vi "Wave2D_Solve QU.vi"(9 "LU of Q":T1, 10 "Q":T3, 11 "U":dbl[][](array[numeric])) -> (0 "error":i32, 3 "Q\\U":dbl[][](array[numeric]))   [LabVIEW 2017, in "NI_PDE.lvlib"]
uses:
  <vilib>/gmath/NI_PDE.lvlib
  <vilib>/Analysis/Matrix/Datatypes/RealMatrix.ctl
  <vilib>/Analysis/7linalg.llb/Solve Linear Equations (multiple right hand).vi
  <vilib>/Analysis/NI_AALPro.lvlib
  <vilib>/Analysis/Matrix/NI_Matrix.lvlib
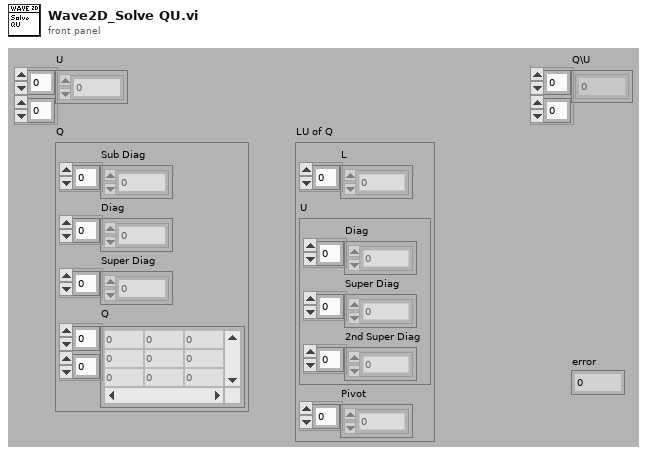
[diagram p1: front panel]
types:
  T1 = cluster{"L":dbl[], "U":cluster{"Diag":dbl[], "Super Diag":dbl[], "2nd Super Diag":dbl[]}, "Pivot":i32[]}
  T2 = typedef "NI_Matrix.lvlib/RealMatrix.ctl" = dbl[][]
  T3 = cluster{"Sub Diag":dbl[], "Diag":dbl[], "Super Diag":dbl[], "Q":T2}
  T4 = cluster{"Diag":dbl[], "Super Diag":dbl[], "2nd Super Diag":dbl[]}
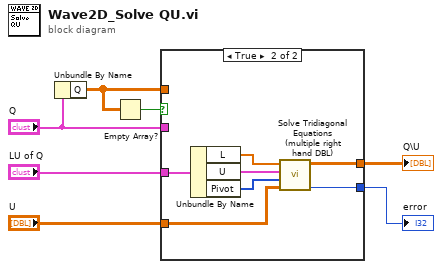
[diagram p0: block diagram]
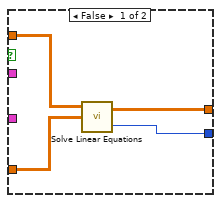
[diagram p2: hidden frame]
diagram:
  n1 = Unbundle By Name("Q") -> ("Q"=w5:T2)
  n2 = Empty Array?(array=w5) -> (empty?=w7:bool)
  n3 = case shown="True" w7 {
    tunnel: "U" -> [w10 w14]
    tunnel: w5 -> [w11 _]
    tunnel: [w9 w13] -> w4
    tunnel: [w8 w12] -> w2
    tunnel: "Q" -> [_ _]
    tunnel: "LU of Q" -> [_ w18]
    frame False {
      n4 = call-poly <vilib>:"Solve Linear Equations.vi"("Known Matrix"=w10, "Input Matrix"=w11) -> ("error"=w8:i32, "Solution Matrix"=w9:T2)  [unwired: 1 in]
    }
    frame True {
      n5 = Unbundle By Name(w18) -> ("L"=w17:dbl[], "U"=w16:T4, "Pivot"=w15:i32[])
      n6 = call <vilib>:"Solve Tridiagonal Equations (multiple right hand DBL).vi"("Known Matrix"=w14, "Pivot"=w15, "U"=w16, "L"=w17) -> ("error"=w12:i32, "Solution Matrix"=w13:T2)  [unwired: 6 out]
    }
  }
  "Q\\U" <- w4
  "error" <- w2
